vi "checkword.vi"(1 "Enable":bool=TRUE) -> (0 "Boolean":bool)   [LabVIEW 2009]
panel:
  # "Subvi that alerts the user for password input"
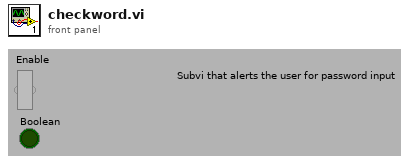
[diagram p1: front panel]
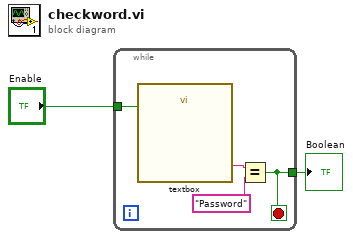
[diagram p0: block diagram]
diagram:
  n1 = while {
    tunnel: [w6] -> w1
    tunnel: "Enable" -> [w3]
    stop <- w6 stop-if-true
    n2 = call "textbox.vi"("Enable"=w3) -> ("word"=w5:string)  [unwired: 16 in, 2 out]
    n3 = Equal?(x=w5, y="Password") -> (x = y?=w6:bool)
  }
  "Boolean" <- w1
